vi "prepare SRQ for axes.vi"(8 "error in (no error)":errorcluster, 10 "category":T1(ring), 11 "GPIB # (in): def. 6":string="6") -> (0 "error out":errorcluster, 3 "GPIB # (out):":string)   [LabVIEW 2017]
doc: "If you want to query the status byte to see if an axis is done moving, you have to send a command like this first, before you send the move command."
uses:
  mc2mc4.llb/MC2/4  SendCommand.VI
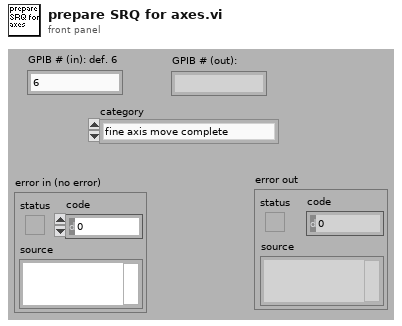
[diagram p1: front panel]
types:
  T1 = enum16{"fine axis move complete", "coarse axis move complete", "either axis move complete", "an axis has reached travel limit"}
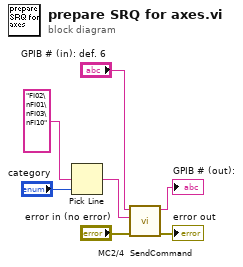
[diagram p0: block diagram]
diagram:
  n1 = Pick Line(multi-line string="FI02\nFI01\nFI03\nFI10", line index="category") -> (output string=w3:string)  [unwired: 1 out]
  n2 = call "MC2/4  SendCommand.VI"("error in (no error)"="error in (no error)", "MC2 / MC4 Command"=w3, "GPIB # (in): def.6"="GPIB # (in): def. 6") -> ("error out"=→"error out":errorcluster, "GPIB # (out)"=→"GPIB # (out):":string)  [unwired: 7 out]
